vi "FestoCPX.DI.Data.State.Get.vi"(8 "error in (no error)":errorcluster, 10 "CPX.DI":T1) -> (0 "error out":errorcluster, 1 "State AND":bool, 2 "State OR":bool, 3 "State":bool, 5 "FrameCounter":i32)   [LabVIEW 2016]
uses:
  FestoCPX.DI.Signal.ctl
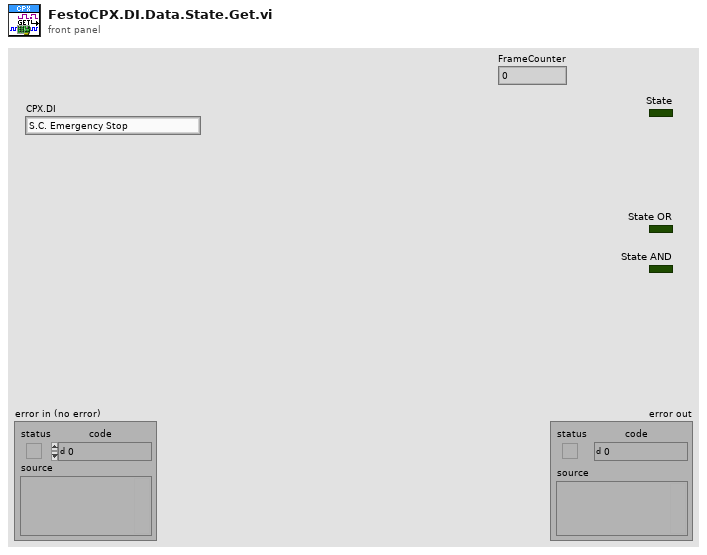
[diagram p1: front panel]
types:
  T1 = typedef "FestoCPX.DI.Signal.ctl" = enum16{"S.C. Emergency Stop", "S.C. Side Door Close", "S.C. Front Door Close", "S.C. Front Door Secured", "Button Start", "Button Stop", "Button Control", "Product Move Home", "Product Move Work", "Table Position", "Table Lock", "Product Lift A Home", "Product Lift B Home", "Product Arm OK", "Product Arm NOK", "Product Arm Work", "Revolver ID 1", "Revolver ID 2", "Revolver ID 3", "Revolver ID 4", "Revolver ID 5", "Air Pressure Inside", "Air Pressure Inlet", "Product Slot 1 A Present", "Product Slot 1 B Present", "Product Slot 2 A Present", "Product Slot 2 B Present", "Product Slot 3 A Present", "Product Slot 3 B Present", "Product Slot 4 A Present", "Product Slot 4 B Present", "Product Final A Present", "Product Final B Present", "Product Output A Present", "Product Output B Present", "Product Container OK Present", "Product Container NOK Present", "Fork ID 1", "Fork ID 2"}
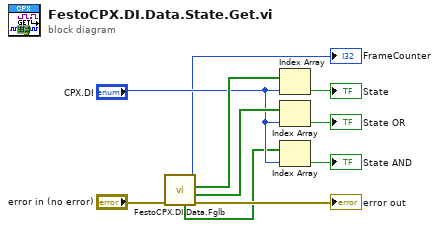
[diagram p0: block diagram]
diagram:
  n1 = call "FestoCPX.DI.Data.Fglb.vi"("error in (no error)"="error in (no error)") -> ("error out"=→"error out":errorcluster, "data OR"=w6:bool[], "data out"=w9:bool[], "FrameCounter"=→"FrameCounter":i32, "data AND"=w2:bool[])  [unwired: 6 in]
  n2 = Index Array(array=w9, index="CPX.DI") -> (element=→"State":bool)
  n3 = Index Array(array=w6, index="CPX.DI") -> (element=→"State OR":bool)
  n4 = Index Array(array=w2, index="CPX.DI") -> (element=→"State AND":bool)
